vi "Envelope(SubVI).vi"(1 "x":dbl[](array[numeric])) -> (0 "Y":dbl[](array[numeric]))   [LabVIEW 2017]
uses:
  <vilib>/Analysis/NI_AALPro.lvlib
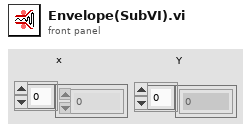
[diagram p1: front panel]
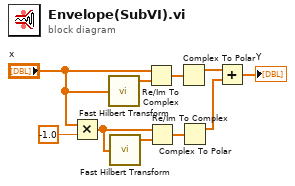
[diagram p0: block diagram]
diagram:
  n1 = Multiply(x="x", y=-1.0) -> (x*y=w4:dbl[])
  n2 = call <vilib>:"Fast Hilbert Transform.vi"("X"="x") -> ("Hilbert{X}"=w10:dbl[])  [unwired: 1 out]
  n3 = call <vilib>:"Fast Hilbert Transform.vi"("X"=w4) -> ("Hilbert{X}"=w8:dbl[])  [unwired: 1 out]
  n4 = Re/Im To Complex(1:w10, 2:"x") -> (0:w9:cdb[])
  n5 = Re/Im To Complex(1:w8, 2:w4) -> (0:w7:cdb[])
  n6 = Complex To Polar(r * e^(i*theta)=w9) -> (r=w3:dbl[])  [unwired: 1 out]
  n7 = Complex To Polar(r * e^(i*theta)=w7) -> (r=w2:dbl[])  [unwired: 1 out]
  n8 = Add(x=w3, y=w2) -> (x+y=→"Y":dbl[])
